vi "MAX_SPRITES.vi"() -> (0 "MAX_SPRITES":u8=20)   [LabVIEW 2020]
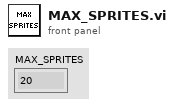
[diagram p1: front panel]
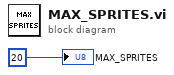
[diagram p0: block diagram]
diagram:
  "MAX_SPRITES" <- u8 20
